vi "LaserCal-Interp.vi"(8 "error in (no error)":errorcluster, 9 "Pulse rate (Hz)":dbl, 10 "Pulse width (us)":dbl, 11 "I-O Data":T1) -> (0 "error out":errorcluster, 3 "Numeric":dbl)   [LabVIEW 2015]
uses:
  Typedefs/LaserCal-Data (PT).ctl
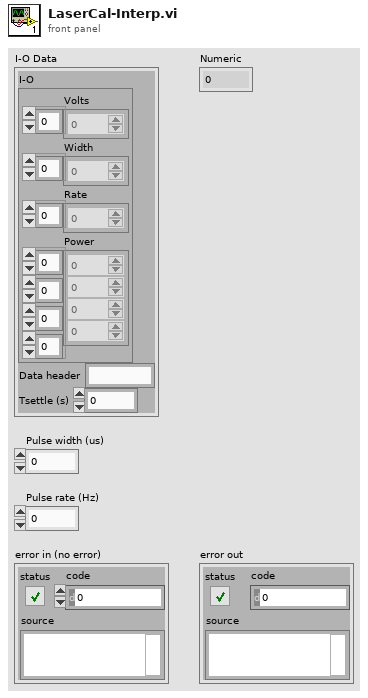
[diagram p1: front panel]
types:
  T1 = typedef "LaserCal-Data (PT).ctl" = cluster{"I-O":cluster{"Volts":dbl[], "Width":dbl[], "Rate":dbl[], "Power":dbl[][][][]}, "Data header":string, "Tsettle (s)":dbl}
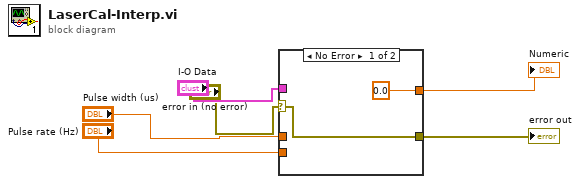
[diagram p0: block diagram]
diagram:
  n1 = case shown="No Error" "error in (no error)" {
    selector: "error in (no error)" -> [w8 _]
    tunnel: [w8 _] -> w2
    tunnel: "Pulse width (us)" -> [_ _]
    tunnel: "Pulse rate (Hz)" -> [_ _]
    tunnel: "I-O Data" -> [_ _]
    tunnel: [0.0 _] -> w6
    frame No Error {
    }
    frame Error {
    }
  }
  "Numeric" <- w6
  "error out" <- w2
